vi "Create Sysdef Tree from Parameters Clusters_Find Channel Ref.vi"(8 "error in (no error)":errorcluster, 10 "hardwareChannel":i32, 11 "Item Ref in":T1 format="%.0x") -> (0 "error out":errorcluster, 2 "Found":bool, 3 "Item Ref out":T1 format="%.0x")   [LabVIEW 2016, in "Ballard Arinc-429 System Explorer.lvlib"]
uses:
  Ballard Arinc-429 System Explorer.lvlib
  Shared/Controls and Global/Global.vi
  Shared/Ballard Arinc-429 Shared.lvlib
  <vilib>/NI Veristand/Custom Device API/Custom Device Item Ref.ctl
  <vilib>/NI VeriStand/Custom Device API/Custom Device API.lvlib
  <vilib>/NI VeriStand/Custom Device Tools/Custom Device Utility Library/Custom Device Utility Library.lvlib
  <vilib>/NI Veristand/Custom Device API/Get Item Property (U16).vi
  <vilib>/NI Veristand/Custom Device Tools/Custom Device Utility Library/NI VeriStand - Search for All Items by GUID.vi
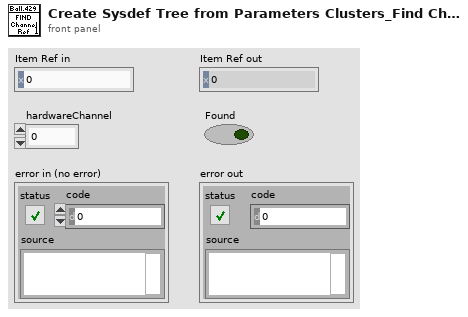
[diagram p1: front panel]
types:
  T1 = typedef "Custom Device API.lvlib/Custom Device Item Ref.ctl" = u64
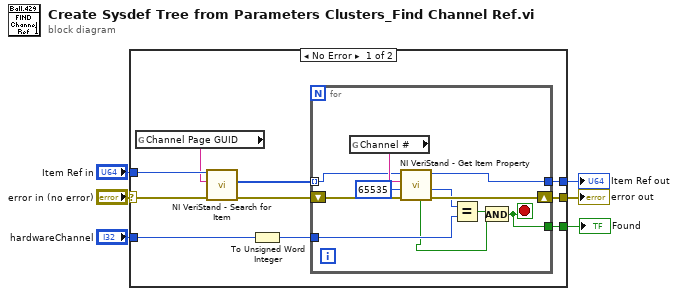
[diagram p0: block diagram]
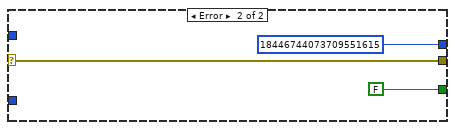
[diagram p2: hidden frame]
diagram:
  n1 = case shown="No Error" "error in (no error)" {
    selector: "error in (no error)" -> [w10 w30]
    tunnel: "hardwareChannel" -> [w16 _]
    tunnel: [w15 T1 18446744073709551615 ("Item Ref")] -> w5
    tunnel: [w14 w30] -> w4
    tunnel: "Item Ref in" -> [w13 _]
    tunnel: [w11 FALSE ("Found")] -> w2
    frame No Error {
      n2 = global read "Global.vi" "Channel Page GUID"() -> (w7:string)
      n3 = call-poly <vilib>:"NI VeriStand - Search for Item.vi"("error in"=w10, "Item GUID"=w7, "Section Ref in"=w13) -> ("error out"=w12:errorcluster, "Item Refs"=w8:T1[])  [unwired: 5 in, 2 out]
      n4 = To Unsigned Word Integer(number=w16) -> (unsigned 16bit integer=w9:u16)
      n5 = for {
        tunnel: w9 -> [w22]
        tunnel: [w26] -> w15
        shift-right: [w25] -> w14
        shift-left: w12 -> [w24]
        tunnel: w8 -> [w20] mode=indexing
        tunnel: [w17] -> w11
        stop <- w17 stop-if-true
        n6 = global read "Global.vi" "Channel #"() -> (w27:string)
        n7 = call-poly <vilib>:"NI VeriStand - Get Item Property.vi"("error in (no error)"=w24, "Default Value"=u16 65535, "Property Name"=w27, "Item Ref in"=w20) -> ("error out"=w25:errorcluster, "Value"=w23:u16, "Item Ref out"=w26:T1, "Found?"=w18:bool)  [unwired: 4 in]
        n8 = Equal?(x=w23, y=w22) -> (x = y?=w19:bool)
        n9 = And(x=w19, y=w18) -> (x .and. y?=w17:bool)
      }
    }
    frame Error {
    }
  }
  "Item Ref out" <- w5
  "error out" <- w4
  "Found" <- w2
